vi "PS35_GetAxisState.vi"(3 "error in (no error)":errorcluster, 4 "Axis number":i32=1 min=0 max=3, 5 "Control unit ID":i32=1 min=1 max=10) -> (0 "error out":errorcluster, 1 "Axis state":i32)   [LabVIEW 2020]
doc: "PS35_GetAxisState.vi, created: 04.03.2009 alex; last change: 22.10.2019 alex;\n\n<B>FUNCTION:</B> \n\nRead axis state.\n----------------------------------------------------------------------------------------\n<B>INPUT:</B>\n[I32] <B>Control unit ID:</B> control unit index. (Default=1, Range=1...10) \n[I32] <B>Axis number:</B> axis number. (Default=1, Range=0...3)\n0 - read state of all axes,\n1...3 - read state of an axis. \n[CLU] <B>error in</B>\n----------------------------------------------------------------------------------------\n<B>OUTPUT:</B>\n[I32] <B>Axis state:</B> state of an axis or all axes.\nAxis number = 0 (all axes)\n0 - any axis is not active,\n1 - any axis is not initialized,\n2 - any axis is switch off,\n3 - all axes are active and initialized and switched on.\nAxis number = 1...3 (an axis)\n0 - axis is not active,\n1 - axis is not initialized,\n2 - axis is switched off,\n3 - axis is active and initialized and switched on.\n[CLU] <B>error out</B>\n----------------------------------------------------------------------------------------\n<B>SUB-VIs:</B>\nPS35_GetReadError.vi\n----------------------------------------------------------------------------------------\n<B>EXT-Calls:</B>\nps35.dll (V2.01)\n----------------------------------------------------------------------------------------"
uses:
  ps35.dll
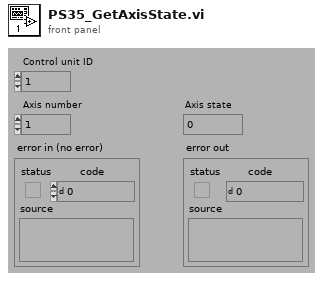
[diagram p1: front panel]
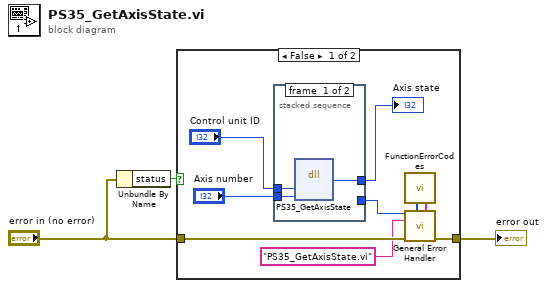
[diagram p0: block diagram]
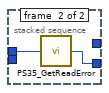
[diagram p2: hidden frame]
diagram:
  n1 = Unbundle By Name("error in (no error)") -> ("status"=w1:bool)
  n2 = case shown="False" w1 {
    tunnel: "error in (no error)" -> [w11 w18]
    tunnel: [w10 w18] -> w3
    frame False {
      n3 = stacked-sequence {
        tunnel: "Control unit ID" -> [w15 w17]
        tunnel: [w14 _] -> w9
        tunnel: [_ w16] -> w8
        tunnel: "Axis number" -> [w13 _]
        frame #0 {
          n4 = dll-call lib="C:/GEECS/Developers Version/source/Device Drivers/OwiSoft_PS35/OWISoftOEM/ps35/labview/lv82/ps35.dll" fn="PS35_GetAxisState" label="PS35_Get\nAxisState"("Index"=w15, "AxisNr"=w13) -> ("Rückgabetyp"=w14:i32)  [unwired: 5 in, 2 out]
        }
        frame #1 {
          n5 = call "PS35_GetReadError.vi"("Control unit ID"=w17) -> ("Read error"=w16:i32)
        }
      }
      "Axis state" <- w9
      n6 = call "FunctionErrorCodes.vi"() -> ("[user-defined codes]"=w5:i32[], "[user-defined descriptions]"=w4:string[])  [unwired: 8 in]
      n7 = call "General Error Handler.vi"("[error code] (0)"=w8, "[user-defined codes]"=w5, "[user-defined descriptions]"=w4, "[error source] (\" \")"="PS35_GetAxisState.vi" ("[error source] (\" \")"), "error in (no error)"=w11) -> ("error out"=w10:errorcluster)  [unwired: 6 in, 4 out]
    }
    frame True {
    }
  }
  "error out" <- w3
